vi "ECC_continuous.vi"() -> ()   [LabVIEW 2013]
uses:
  ecc_continuous_sm.ctl
  <vilib>/DAQmx/write.llb/DAQmx Write (Analog Wfm 1Chan NSamp).vi
  <vilib>/DAQmx/create/channels.llb/DAQmx Create Channel (AO-Voltage-Basic).vi
  <vilib>/DAQmx/configure/timing.llb/DAQmx Timing (Use Waveform).vi
  <vilib>/DAQmx/miscellaneous.llb/DAQmx Fill In Error Info.vi
panel:
  in  "StopSweep":bool
  in  "R&S/5181":bool=TRUE
  in  "T_sweep, s":dbl min=0.0 step=0.001 format="%#_6f"
  in  "N_steps":i32 min=0 step=1
  in  "Waveform":T1(ring)
  in  "A, mV":i32=10
  in  "fm, kHz":i32=400 step=1
  in  "f0, MHz":dbl=32.7 min=0.0 step=0.001 format="%#_6f"
  out "APS_off_status":bool=TRUE
  out "R&S_off_status":bool=TRUE
  in  "Use_APS":bool=TRUE
  out "DAC_status":bool
  out "RF_status":bool
  out "APS_status":bool
  in  "APS address":refnum<visa-resource-name>="COM3"
  in  "Init Devices":bool
  in  "StartSweep":bool
  in  "Exit":bool
  in  "DAC channel":tag="Dev1/ao0"
  in  "RF address":string(combo)="19"
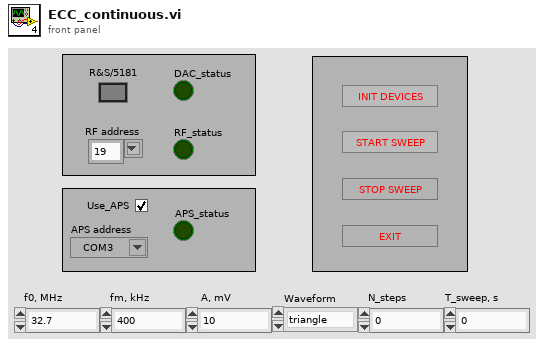
[diagram p1: front panel]
types:
  T1 = enum16{"triangle", "saw_direct", "saw_invert", "sine"}
  T2 = typedef "ecc_continuous_sm.ctl" = enum16{"idle", "init_daq", "init_rf", "init_ps", "rf_set", "set_wf", "rf_on", "ps_on", "daq_start", "ps_off", "rf_off", "daq_stop", "exit"}
  T3 = enum8{"Enabled", "Disabled", "Disabled and Grayed Out"}
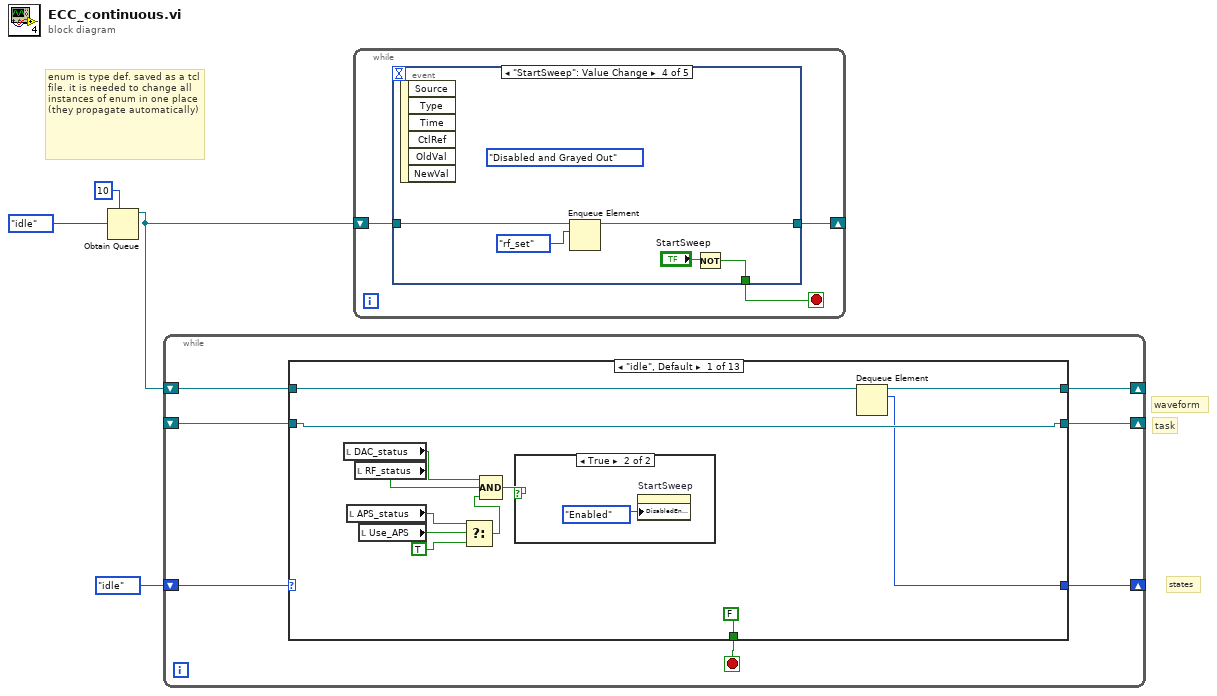
[diagram p0: block diagram]
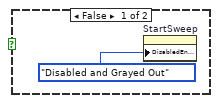
[diagram p2: hidden frame]
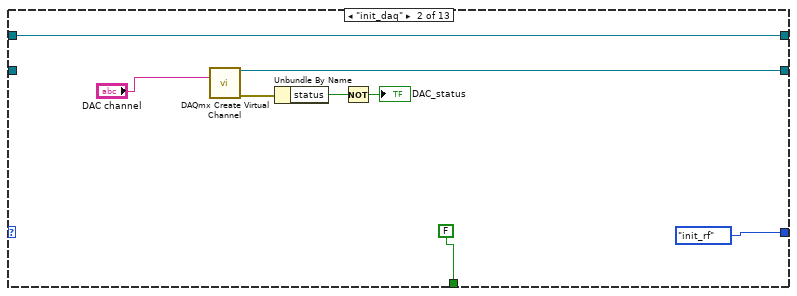
[diagram p3: hidden frame]
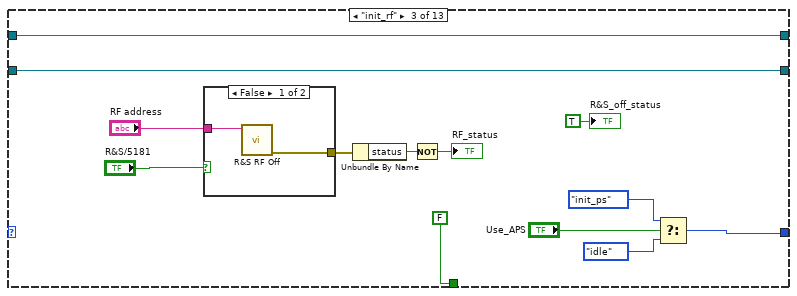
[diagram p4: hidden frame]
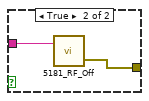
[diagram p5: hidden frame]
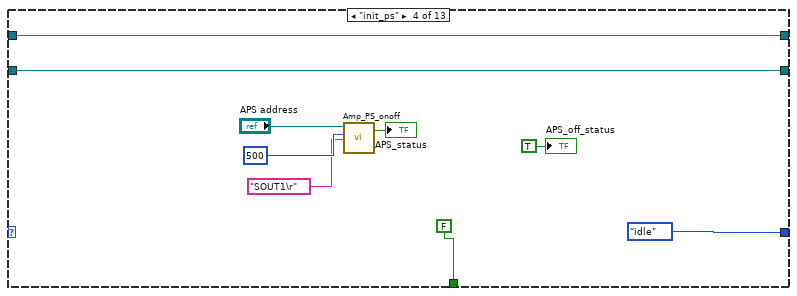
[diagram p6: hidden frame]
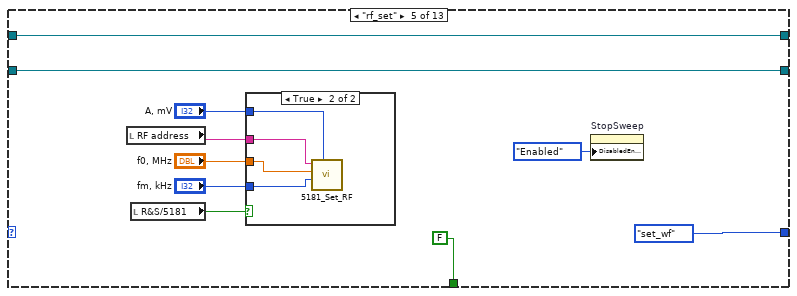
[diagram p7: hidden frame]
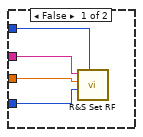
[diagram p8: hidden frame]
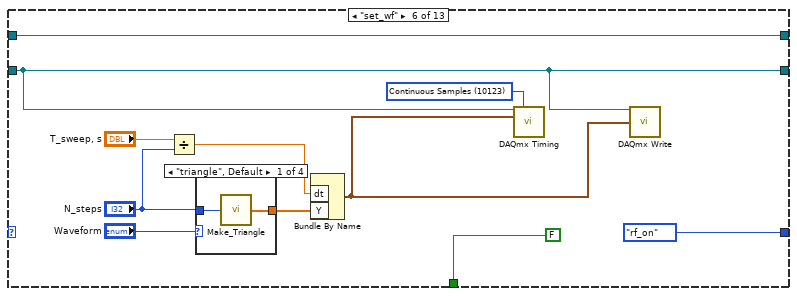
[diagram p9: hidden frame]
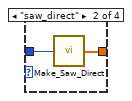
[diagram p10: hidden frame]
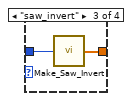
[diagram p11: hidden frame]
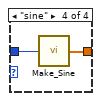
[diagram p12: hidden frame]
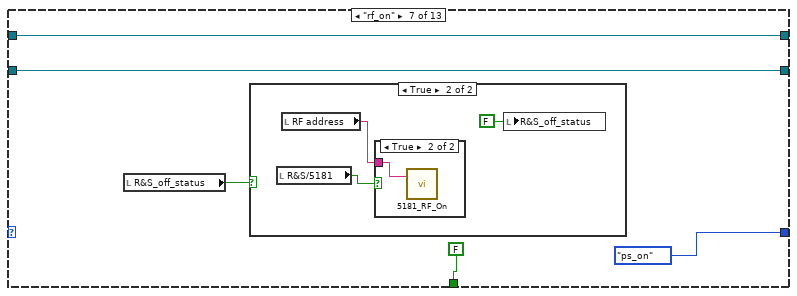
[diagram p13: hidden frame]
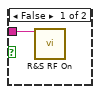
[diagram p15: hidden frame]
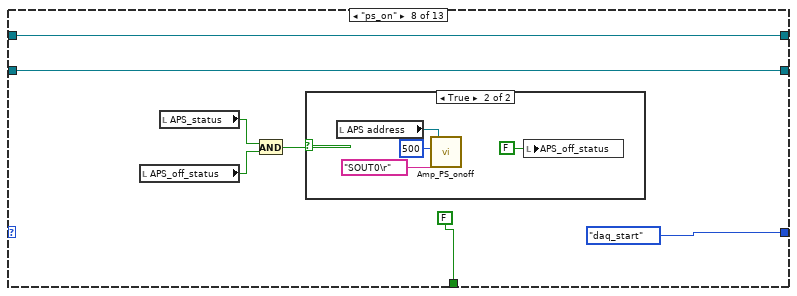
[diagram p16: hidden frame]
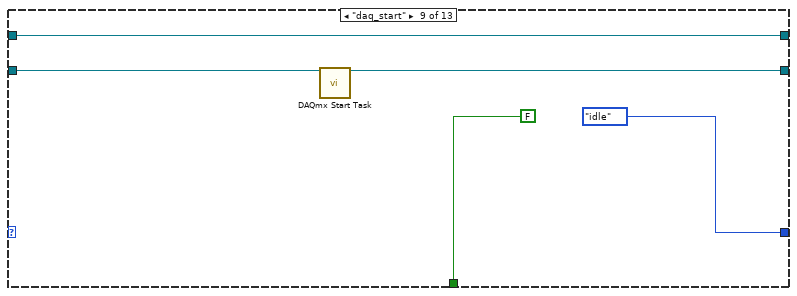
[diagram p18: hidden frame]
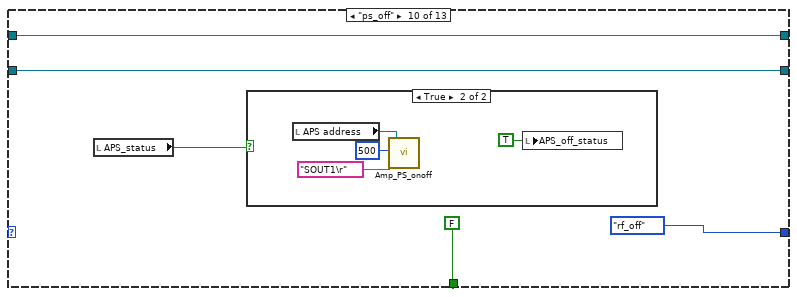
[diagram p19: hidden frame]
diagram:
  # "enum is type def. saved as a tcl file. it is needed to change all instances of enum in one place (they propagate automatically)"
  # "states"
  # "waveform"
  # "task"
  n1 = Obtain Queue(max queue size (-1, unlimited)=10, element data type=ecc_continuous_sm."idle" ("Enum")) -> (queue out=w3:refnum<queue>)  [unwired: 3 in, 2 out]
  n2 = while {
    shift-right: [w9] -> _
    shift-left: ecc_continuous_sm."idle" ("Enum") -> [w5]
    shift-right: [w11] -> _
    shift-left: _ -> [w10]
    shift-right: [w7] -> _
    shift-left: w3 -> [w8]
    stop <- w6 stop-if-true
    n3 = case shown="\"idle\", Default" w5 {
      selector: w5 -> [_ _ _ _ _ _ _ _ _ _ _ _ w155]
      tunnel: [w23 w32 w46 w59 w68 w80 w100 w113 w121 w127 w137 w144 w152] -> w11
      tunnel: w10 -> [w23 _ w46 w59 w68 w80 w100 w113 w122 w127 w137 w145 w152]
      tunnel: [w20 ecc_continuous_sm."init_rf" ("Enum") w40 ecc_continuous_sm."idle" ("Enum") ecc_continuous_sm."set_wf" ("Enum") ecc_continuous_sm."rf_on" ("Enum") ecc_continuous_sm."ps_on" ("Enum") ecc_continuous_sm."daq_start" ("Enum") ecc_continuous_sm."idle" ("Enum") ecc_continuous_sm."rf_off" ("Enum") ecc_continuous_sm."daq_stop" ("Enum") ecc_continuous_sm."idle" ("Enum") w155] -> w9
      tunnel: w8 -> [w22 w30 w44 w57 w66 w86 w101 w111 w119 w125 w138 w142 w154]
      tunnel: [w21 w30 w44 w57 w66 w86 w101 w111 w119 w125 w138 w142 w154] -> w7
      tunnel: [FALSE FALSE FALSE FALSE FALSE FALSE FALSE FALSE FALSE FALSE FALSE FALSE TRUE] -> w6
      frame "idle", Default {
        n4 = local read "DAC_status"() -> (w18:bool)
        n5 = local read "APS_status"() -> (w12:bool)
        n6 = local read "RF_status"() -> (w17:bool)
        n7 = local read "Use_APS"() -> (w16:bool)
        n8 = Select(t=w12, s=w16, f=TRUE) -> (s? t:f=w14:bool)
        n9 = Compound Arithmetic op=AND(w18, w17, w14) -> (w13:bool)
        n10 = case shown="True" w13 {
          frame False {
            n11 = property on="StartSweep" class="Bool"("DisabledEnum"=T3."Disabled and Grayed Out" ("Disabled")) -> ()  [unwired: 2 in, 2 out]
          }
          frame True {
            n12 = property on="StartSweep" class="Bool"("DisabledEnum"=T3."Enabled" ("Disabled")) -> ()  [unwired: 2 in, 2 out]
          }
        }
        n13 = Dequeue Element(queue=w22) -> (queue out=w21:refnum<queue>, element=w20:T2)  [unwired: 2 in, 2 out]
      }
      frame "init_daq" {
        n14 = call-poly <vilib>:"DAQmx Create Virtual Channel.vi"("physical channels"="DAC channel") -> ("task out"=w32:refnum<k21>, "error out"=w29:errorcluster)  [unwired: 13 in]
        n15 = Unbundle By Name(w29) -> ("status"=w28:bool)
        n16 = Not(x=w28) -> (.not. x?=→"DAC_status":bool)
      }
      frame "init_rf" {
        n17 = case shown="False" "R&S/5181" {
          tunnel: "RF address" -> [w48 w50]
          tunnel: [w47 w49] -> w37
          frame False {
            n18 = call "R&S RF Off.vi"("address"=w48) -> ("error out"=w47:errorcluster)  [unwired: 5 in, 1 out]
          }
          frame True {
            n19 = call "5181_RF_Off.vi"("address"=w50) -> ("error out"=w49:errorcluster)  [unwired: 1 in, 1 out]
          }
        }
        n20 = Unbundle By Name(w37) -> ("status"=w42:bool)
        n21 = Not(x=w42) -> (.not. x?=→"RF_status":bool)
        n22 = Select(t=ecc_continuous_sm."init_ps" ("Enum"), s="Use_APS", f=ecc_continuous_sm."idle" ("Enum")) -> (s? t:f=w40:T2)
        "R&S_off_status" <- TRUE ("R&S_off_status")
      }
      frame "init_ps" {
        n23 = call "Amp_PS_onoff.vi"("On/Off Control"="SOUT1\r", "delay before read (ms)"=u32 500, "Amp PS address"="APS address") -> ("status"=→"APS_status":bool)  [unwired: 1 in, 1 out]
        "APS_off_status" <- TRUE ("APS_off_status")
      }
      frame "rf_set" {
        n24 = local read "RF address"() -> (w69:string)
        n25 = local read "R&S/5181"() -> (w62:bool)
        n26 = case shown="True" w62 {
          tunnel: w69 -> [w73 w77]
          tunnel: "A, mV" -> [w72 w76]
          tunnel: "f0, MHz" -> [w71 w75]
          tunnel: "fm, kHz" -> [w70 w74]
          frame False {
            n27 = call "R&S Set RF.vi"("amplitude (mV)"=w72, "modulation (kHz)"=w70, "center frequency (MHz)"=w71, "address"=w73) -> ()  [unwired: 3 in, 2 out]
          }
          frame True {
            n28 = call "5181_Set_RF.vi"("address"=w77, "center frequency (MHz)"=w75, "modulation (kHz)"=w74, "amplitude (mV)"=w76) -> ()  [unwired: 1 in, 2 out]
          }
        }
        n29 = property on="StopSweep" class="Bool"("DisabledEnum"=T3."Enabled" ("Disabled")) -> ()  [unwired: 2 in, 2 out]
      }
      frame "set_wf" {
        w81 = 10123 items=["Finite Samples"=10178, "Continuous Samples"=10123, "Hardware Timed Single Point"=12522] ("sample mode")
        n30 = Divide(x="T_sweep, s", y="N_steps") -> (x/y=w88:dbl)
        n31 = case shown="\"triangle\", Default" "Waveform" {
          tunnel: [w90 w92 w94 w96] -> w82
          tunnel: "N_steps" -> [w89 w91 w93 w95]
          frame "triangle", Default {
            n32 = call "Make_Triangle.vi"("N_steps_1"=w89) -> ("TriangleWaveform"=w90:dbl[])
          }
          frame "saw_direct" {
            n33 = call "Make_Saw_Direct.vi"("N_steps_1"=w91) -> ("SawDirectWaveform"=w92:dbl[])
          }
          frame "saw_invert" {
            n34 = call "Make_Saw_Invert.vi"("N_steps_1"=w93) -> ("SawInvertWaveform"=w94:dbl[])
          }
          frame "sine" {
            n35 = call "Make_Sine.vi"("N_steps_1"=w95) -> ("SineWaveform"=w96:dbl[])
          }
        }
        n36 = Bundle By Name("dt"=w88, "Y"=w82) -> (w79:waveform(dbl))  [unwired: 1 in]
        n37 = call-poly <vilib>:"DAQmx Timing.vi"("task/channels in"=w80, "sample mode"=w81, "waveform"=w79) -> ()  [unwired: 11 in, 2 out]
        n38 = call-poly <vilib>:"DAQmx Write.vi"("task/channels in"=w80, "data"=w79) -> ()  [unwired: 11 in, 3 out]
      }
      frame "rf_on" {
        n39 = local read "R&S_off_status"() -> (w97:bool)
        n40 = case shown="True" w97 {
          frame False {
          }
          frame True {
            n41 = local read "R&S/5181"() -> (w102:bool)
            n42 = local read "RF address"() -> (w104:string)
            n43 = case shown="True" w102 {
              tunnel: w104 -> [w105 w106]
              frame False {
                n44 = call "R&S RF On.vi"("address"=w105) -> ()  [unwired: 5 in, 2 out]
              }
              frame True {
                n45 = call "5181_RF_On.vi"("address"=w106) -> ()  [unwired: 1 in, 2 out]
              }
            }
            n46 = local write "R&S_off_status"(FALSE ("R&S_off_status")) -> ()
          }
        }
      }
      frame "ps_on" {
        n47 = local read "APS_off_status"() -> (w110:bool)
        n48 = local read "APS_status"() -> (w108:bool)
        n49 = And(x=w108, y=w110) -> (x .and. y?=w109:bool)
        n50 = case shown="True" w109 {
          frame False {
          }
          frame True {
            n51 = local read "APS address"() -> (w114:refnum<visa-resource-name>)
            n52 = call "Amp_PS_onoff.vi"("On/Off Control"="SOUT0\r", "delay before read (ms)"=u32 500, "Amp PS address"=w114) -> ()  [unwired: 1 in, 2 out]
            n53 = local write "APS_off_status"(FALSE ("APS_off_status")) -> ()
          }
        }
      }
      frame "daq_start" {
        n54 = call <vilib>:"DAQmx Start Task.vi"("task/channels in"=w122) -> ("task out"=w121:refnum<k21>)  [unwired: 13 in, 1 out]
      }
      frame "ps_off" {
        n55 = local read "APS_status"() -> (w123:bool)
        n56 = case shown="True" w123 {
          frame False {
          }
          frame True {
            n57 = local read "APS address"() -> (w128:refnum<visa-resource-name>)
            n58 = call "Amp_PS_onoff.vi"("On/Off Control"="SOUT1\r", "delay before read (ms)"=u32 500, "Amp PS address"=w128) -> ()  [unwired: 1 in, 2 out]
            n59 = local write "APS_off_status"(TRUE ("APS_off_status")) -> ()
          }
        }
      }
      frame "rf_off" {
        n60 = local read "RF address"() -> (w135:string)
        n61 = local read "R&S/5181"() -> (w133:bool)
        n62 = case shown="True" w133 {
          tunnel: w135 -> [w139 w140]
          frame False {
            n63 = call "R&S RF Off.vi"("address"=w139) -> ()  [unwired: 5 in, 2 out]
          }
          frame True {
            n64 = call "5181_RF_Off.vi"("address"=w140) -> ()  [unwired: 1 in, 2 out]
          }
        }
        n65 = local write "R&S_off_status"(TRUE ("R&S_off_status")) -> ()
      }
      frame "daq_stop" {
        n66 = call <vilib>:"DAQmx Stop Task.vi"("task/channels in"=w145) -> ("task out"=w144:refnum<k21>)  [unwired: 13 in, 1 out]
      }
      frame "exit" {
        w148 = FALSE ("DAC_status")
        n67 = local read "APS address"() -> (w150:refnum<visa-resource-name>)
        n68 = local read "Use_APS"() -> (w151:bool)
        n69 = case shown="True" w151 {
          tunnel: w150 -> [_ w158]
          frame False {
          }
          frame True {
            n70 = call "Amp_PS_onoff.vi"("On/Off Control"="SOUT1\r", "delay before read (ms)"=u32 50, "Amp PS address"=w158) -> ()  [unwired: 1 in, 2 out]
          }
        }
        n71 = local read "RF address"() -> (w147:string)
        n72 = local read "R&S/5181"() -> (w146:bool)
        n73 = case shown="True" w146 {
          tunnel: w147 -> [w156 w157]
          frame False {
            n74 = call "R&S RF Off.vi"("address"=w156) -> ()  [unwired: 5 in, 2 out]
          }
          frame True {
            n75 = call "5181_RF_Off.vi"("address"=w157) -> ()  [unwired: 1 in, 2 out]
          }
        }
        n76 = local write "DAC_status"(w148) -> ()
        n77 = local write "RF_status"(w148) -> ()
        n78 = local write "APS_status"(w148) -> ()
        n79 = property on="Init Devices" class="Bool"("DisabledEnum"=T3."Enabled" ("Disabled")) -> ()  [unwired: 2 in, 2 out]
      }
    }
  }
  n80 = while {
    shift-right: [w161] -> _
    shift-left: w3 -> [w162]
    stop <- w163 stop-if-true
    n81 = event shown="[3] \"StartSweep\": Value Change" {
      selector: _ -> [_ _ _ _ _]
      dyn-events: _ -> [_ _ _ _ _]
      timeout: _ -> [_ _ _ _ _]
      tunnel: [_ "Exit" w173 w178 w185] -> w163
      tunnel: w162 -> [w164 w167 w172 w177 w183]
      tunnel: [w164 w166 w171 w176 w182] -> w161
      event Timeout {
        n82 = event-data() -> ()  [unwired: 1 in, 3 out]
      }
      event "Exit": Value Change {
        n83 = event-data() -> ()  [unwired: 1 in, 6 out]
        n84 = Enqueue Element(queue=w167, element=ecc_continuous_sm."exit" ("Enum")) -> (queue out=w166:refnum<queue>)  [unwired: 2 in, 2 out]
      }
      event "Init Devices": Value Change {
        n85 = event-data() -> ()  [unwired: 1 in, 6 out]
        n86 = Enqueue Element(queue=w172, element=ecc_continuous_sm."init_daq" ("Enum")) -> (queue out=w171:refnum<queue>)  [unwired: 2 in, 2 out]
        n87 = property on="Init Devices" class="Bool"("DisabledEnum"=T3."Disabled and Grayed Out" ("Disabled")) -> ()  [unwired: 2 in, 2 out]
        n88 = Not(x="Init Devices") -> (.not. x?=w173:bool)
      }
      event "StartSweep": Value Change {
        (unwired) T3."Disabled and Grayed Out" ("Disabled")
        n89 = event-data() -> ()  [unwired: 1 in, 6 out]
        n90 = Enqueue Element(queue=w177, element=ecc_continuous_sm."rf_set" ("Enum")) -> (queue out=w176:refnum<queue>)  [unwired: 2 in, 2 out]
        n91 = Not(x="StartSweep") -> (.not. x?=w178:bool)
      }
      event "StopSweep": Value Change {
        n92 = event-data() -> ()  [unwired: 1 in, 6 out]
        n93 = Enqueue Element(queue=w183, element=ecc_continuous_sm."ps_off" ("Enum")) -> (queue out=w182:refnum<queue>)  [unwired: 2 in, 2 out]
        n94 = property on="StopSweep" class="Bool"("DisabledEnum"=T3."Disabled" ("Disabled")) -> ()  [unwired: 2 in, 2 out]
        n95 = Not(x="StopSweep") -> (.not. x?=w185:bool)
      }
    }
  }
